vi "CRYInit Listbox.vi"(9 "Pane 2":refnum<vi>, 10 "Splitter":refnum<vi>, 11 "Pane 1":refnum<vi>) -> ()   [LabVIEW 2013]
uses:
  <vilib>/Utility/miscctls.llb/LVPositionTypeDef.ctl
  Global/CRYCurve Library Global.vi
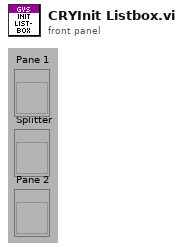
[diagram p1: front panel]
types:
  T1 = typedef "LVPositionTypeDef.ctl" = cluster{"Left":i32, "Top":i32}
  T2 = typedef "LVRectTypeDef.ctl" = cluster{"Left":i16, "Top":i16, "Right":i16, "Bottom":i16}
  T3 = typedef "LVBoundsTypeDef.ctl" = cluster{"Width":u32, "Height":u32}
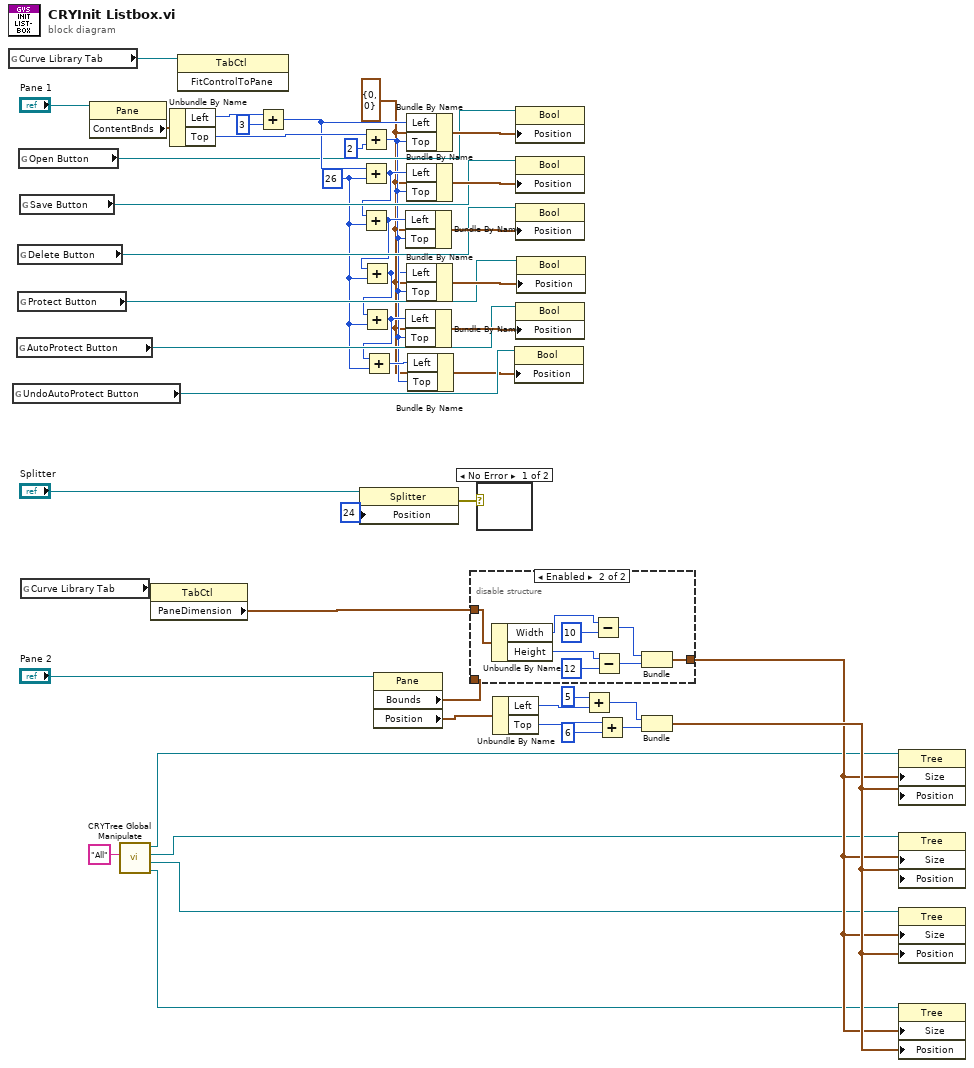
[diagram p0: block diagram]
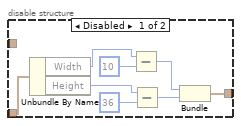
[diagram p2: hidden frame]
diagram:
  w24 = i16 26 ("y")
  w2 = T1 {"Left"=0, "Top"=0} ("Position")
  n1 = global read "CRYCurve Library Global.vi" "Curve Library Tab"() -> (w38:refnum<vi>)
  n2 = global read "CRYCurve Library Global.vi" "UndoAutoProtect Button"() -> (w31:refnum<vi>)
  n3 = global read "CRYCurve Library Global.vi" "AutoProtect Button"() -> (w27:refnum<vi>)
  n4 = global read "CRYCurve Library Global.vi" "Delete Button"() -> (w35:refnum<vi>)
  n5 = global read "CRYCurve Library Global.vi" "Protect Button"() -> (w34:refnum<vi>)
  n6 = global read "CRYCurve Library Global.vi" "Open Button"() -> (w37:refnum<vi>)
  n7 = global read "CRYCurve Library Global.vi" "Save Button"() -> (w36:refnum<vi>)
  n8 = global read "CRYCurve Library Global.vi" "Curve Library Tab"() -> (w4:refnum<vi>)
  n9 = property class="Pane"(reference="Pane 1") -> ("ContentBnds"=w49:T2)  [unwired: 1 in, 2 out]
  n10 = call "CRYTree Global Manipulate.vi"("sOption"="All") -> ("WFM Tree"=w6:refnum<vi>, "Results Tree"=w7:refnum<vi>, "Values Tree"=w8:refnum<vi>, "Tree/Curve Tree"=w9:refnum<vi>)  [unwired: 7 in]
  n11 = property class="TabCtl"(reference=w4) -> ("PaneDimension"=w3:T3)  [unwired: 1 in, 2 out]
  n12 = Unbundle By Name(w49) -> ("Left"=w39:i16, "Top"=w44:i16)
  n13 = invoke class="TabCtl" method="FitControlToPane"(reference=w38) -> ()  [unwired: 2 in, 3 out]
  n14 = Add(x=w39, y=i16 3) -> (x+y=w41:i16)
  n15 = property on="Property Node" class="Splitter"(reference="Splitter", "Position"=24 ("Splitter Position")) -> (error out=w11:errorcluster)  [unwired: 1 in, 1 out]
  n16 = Add(x=w44, y=i16 2) -> (x+y=w25:i16)
  n17 = Add(x=w41, y=w24) -> (x+y=w33:i16)
  n18 = Add(x=w33, y=w24) -> (x+y=w32:i16)
  n19 = Add(x=w32, y=w24) -> (x+y=w1:i16)
  n20 = Add(x=w1, y=w24) -> (x+y=w26:i16)
  n21 = Add(x=w26, y=w24) -> (x+y=w29:i16)
  n22 = property class="Pane"(reference="Pane 2") -> ("Bounds"=w17:T3, "Position"=w16:T1)  [unwired: 1 in, 2 out]
  n23 = Bundle By Name(cluster=w2, "Left"=w32, "Top"=w25) -> (w45:T1)
  n24 = Bundle By Name(cluster=w2, "Left"=w26, "Top"=w25) -> (w28:T1)
  n25 = Bundle By Name(cluster=w2, "Left"=w41, "Top"=w25) -> (w48:T1)
  n26 = Bundle By Name(cluster=w2, "Left"=w33, "Top"=w25) -> (w46:T1)
  n27 = Bundle By Name(cluster=w2, "Left"=w1, "Top"=w25) -> (w42:T1)
  n28 = Bundle By Name(cluster=w2, "Left"=w29, "Top"=w25) -> (w30:T1)
  n29 = disable-structure shown="Enabled" {
    disable-tunnel: w17 -> [w52 _]
    disable-tunnel: [w51 w60] -> w13
    disable-tunnel: w3 -> [_ w58]
    frame Disabled {
      n30 = Unbundle By Name(w52) -> ("Width"=w53:u32, "Height"=w54:u32)
      n31 = Subtract(x=w53, y=u32 10) -> (x-y=w56:u32)
      n32 = Subtract(x=w54, y=u32 36) -> (x-y=w57:u32)
      n33 = Bundle(w56, w57) -> (w51:cluster{u32, u32})  [unwired: 1 out]
    }
    frame Enabled {
      n34 = Unbundle By Name(w58) -> ("Width"=w61:u32, "Height"=w62:u32)
      n35 = Subtract(x=w61, y=u32 10) -> (x-y=w64:u32)
      n36 = Subtract(x=w62, y=u32 12) -> (x-y=w65:u32)
      n37 = Bundle(w64, w65) -> (w60:cluster{u32, u32})  [unwired: 1 out]
    }
  }
  n38 = case shown="No Error" w11 {
    frame No Error {
    }
    frame Error {
    }
  }
  n39 = Unbundle By Name(w16) -> ("Left"=w18:i32, "Top"=w21:i32)
  n40 = property class="Bool"(reference=w31, "Position"=w30) -> ()  [unwired: 1 in, 2 out]
  n41 = property on="Property Node" class="Bool"(reference=w37, "Position"=w48) -> ()  [unwired: 1 in, 2 out]
  n42 = property on="Property Node" class="Bool"(reference=w36, "Position"=w46) -> ()  [unwired: 1 in, 2 out]
  n43 = property on="Property Node" class="Bool"(reference=w35, "Position"=w45) -> ()  [unwired: 1 in, 2 out]
  n44 = property on="Property Node" class="Bool"(reference=w27, "Position"=w28) -> ()  [unwired: 1 in, 2 out]
  n45 = property on="Property Node" class="Bool"(reference=w34, "Position"=w42) -> ()  [unwired: 1 in, 2 out]
  n46 = Add(x=5, y=w18) -> (x+y=w22:i32)
  n47 = Add(x=w21, y=6) -> (x+y=w20:i32)
  n48 = Bundle(w22, w20) -> (w14:cluster{i32, i32})  [unwired: 1 out]
  n49 = property on="Property Node" class="Tree"(reference=w9, "Size"=w13, "Position"=w14) -> ()  [unwired: 1 in, 2 out]
  n50 = property on="Property Node" class="Tree"(reference=w8, "Size"=w13, "Position"=w14) -> ()  [unwired: 1 in, 2 out]
  n51 = property on="Property Node" class="Tree"(reference=w7, "Size"=w13, "Position"=w14) -> ()  [unwired: 1 in, 2 out]
  n52 = property on="Property Node" class="Tree"(reference=w6, "Size"=w13, "Position"=w14) -> ()  [unwired: 1 in, 2 out]
